vi "AOL Z Cal load-Init globals.vi"   [LabVIEW 2020]
uses:
  Configuration code/Calibration/Globals/gl_Calibration globals.vi
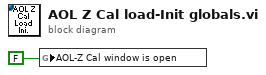
[diagram p0: block diagram]
diagram:
  n1 = global write "gl_Calibration globals.vi" "AOL-Z Cal window is open"(FALSE ("Bring to front")) -> ()
